vi "Intellirupter2.vi"() -> ()   [LabVIEW 2016]
uses:
  <vilib>/rvi/Emulation/niFpgaGetClockAttributes.vi
  <vilib>/rvi/Emulation/niFpgaSctlEmulationGetInTimedLoop.vi
  <vilib>/rvi/Emulation/niFpgaEmulationReportErrorSimple.vi
  <vilib>/rvi/eio/common/nirviEmuTemplateMethod_errors.vi
  <vilib>/rvi/interface/RandomDataEmulation/niFpgaRandomDataHandleErrors.vi
  <vilib>/rvi/Emulation/niFpgaCriticalErrorInLSC.vi
  <vilib>/eio/EIONode/EIONode.xnode
  <vilib>/rvi/DataTransferAndStorage/Container/XNode/niFpgaContainer.xnode
  <vilib>/rvi/interface/RandomDataEmulation/nirviRandomDataFpgaReadWriteTemplate.vi
panel:
  in  "Stop":bool
  in  "Loop Rate (uS)":u32
  out "Data FIFO Full":bool
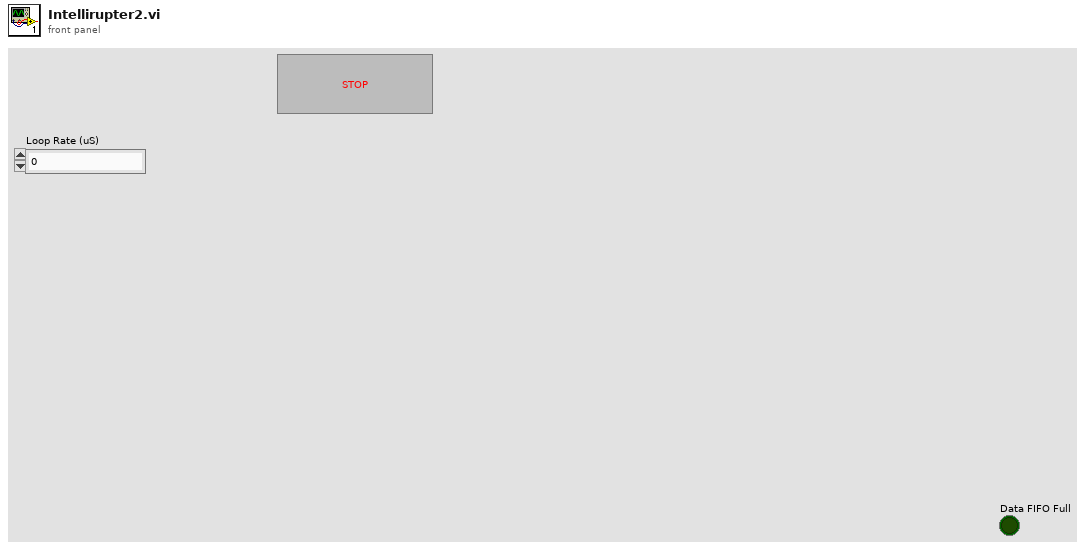
[diagram p1: front panel]
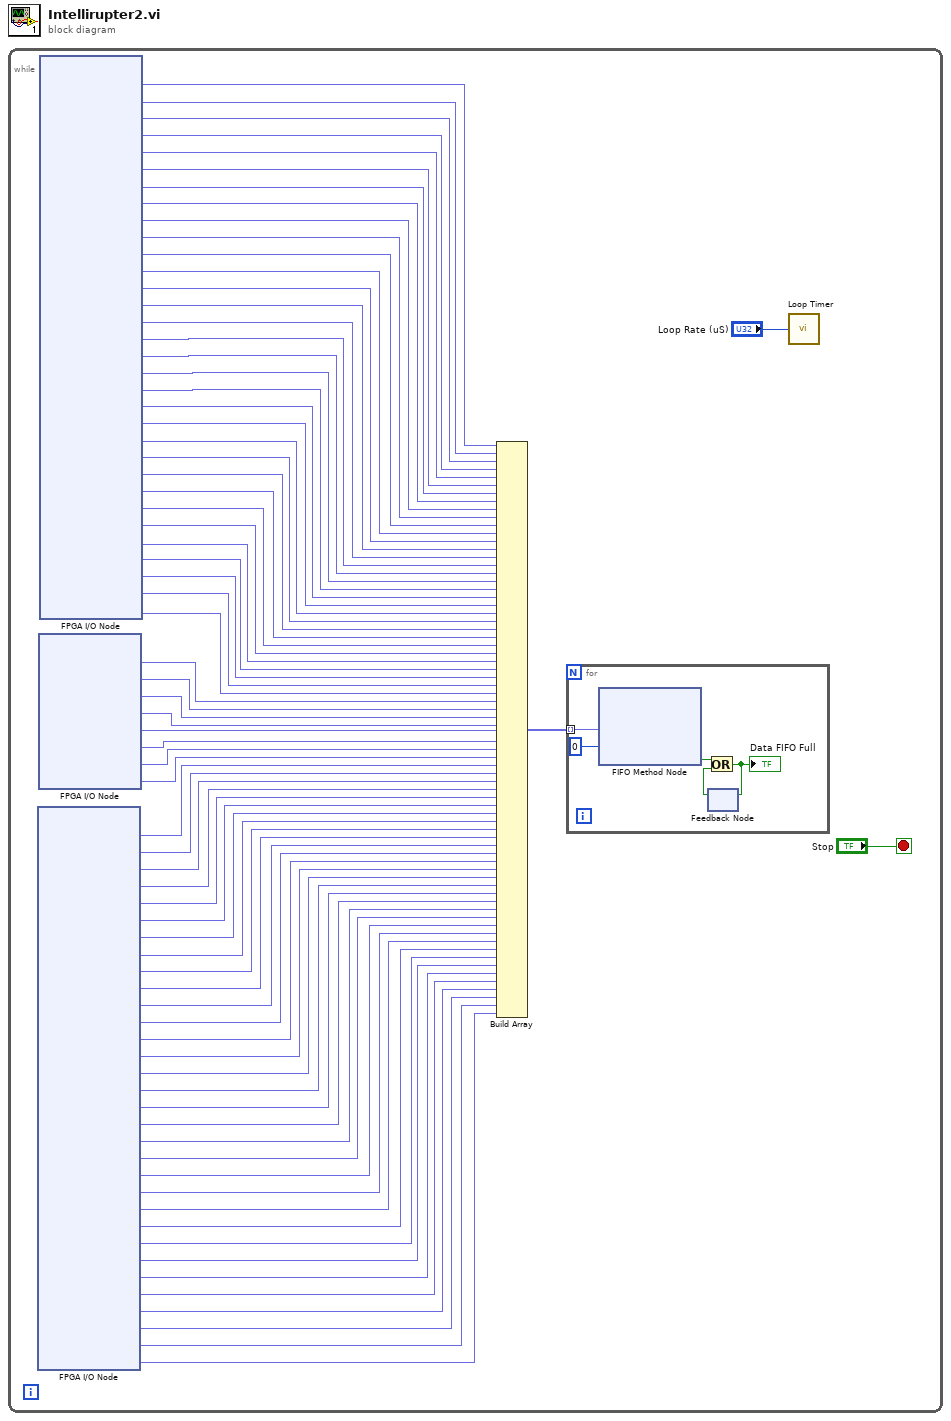
[diagram p0: block diagram]
diagram:
  n1 = while {
    stop <- "Stop" stop-if-true
    n2 = xnode "FPGA I/O Node"() -> ("Mod8/AI0"=w33:fxp<+/-,26,5>, "Mod8/AI1"=w32:fxp<+/-,26,5>, "Mod8/AI2"=w31:fxp<+/-,26,5>, "Mod8/AI3"=w30:fxp<+/-,26,5>, "Mod8/AI4"=w29:fxp<+/-,26,5>, "Mod8/AI5"=w28:fxp<+/-,26,5>, "Mod8/AI6"=w27:fxp<+/-,26,5>, "Mod8/AI7"=w26:fxp<+/-,26,5>, "Mod8/AI8"=w25:fxp<+/-,26,5>, "Mod8/AI9"=w24:fxp<+/-,26,5>, "Mod8/AI10"=w23:fxp<+/-,26,5>, "Mod8/AI11"=w22:fxp<+/-,26,5>, "Mod8/AI12"=w21:fxp<+/-,26,5>, "Mod8/AI13"=w20:fxp<+/-,26,5>, "Mod8/AI14"=w19:fxp<+/-,26,5>, "Mod8/AI15"=w18:fxp<+/-,26,5>, "Mod8/AI16"=w17:fxp<+/-,26,5>, "Mod8/AI17"=w16:fxp<+/-,26,5>, "Mod8/AI18"=w15:fxp<+/-,26,5>, "Mod8/AI19"=w14:fxp<+/-,26,5>, "Mod8/AI20"=w13:fxp<+/-,26,5>, "Mod8/AI21"=w12:fxp<+/-,26,5>, "Mod8/AI22"=w11:fxp<+/-,26,5>, "Mod8/AI23"=w10:fxp<+/-,26,5>, "Mod8/AI24"=w9:fxp<+/-,26,5>, "Mod8/AI25"=w8:fxp<+/-,26,5>, "Mod8/AI26"=w7:fxp<+/-,26,5>, "Mod8/AI27"=w6:fxp<+/-,26,5>, "Mod8/AI28"=w5:fxp<+/-,26,5>, "Mod8/AI29"=w4:fxp<+/-,26,5>, "Mod8/AI30"=w3:fxp<+/-,26,5>, "Mod8/AI31"=w2:fxp<+/-,26,5>)  [unwired: 32 in, 32 out]
    n3 = xnode "FPGA I/O Node"() -> ("Mod5/AI20"=w41:fxp<+/-,26,5>, "Mod5/AI1"=w40:fxp<+/-,26,5>, "Mod5/AI2"=w39:fxp<+/-,26,5>, "Mod5/AI3"=w38:fxp<+/-,26,5>, "Mod5/AI0"=w37:fxp<+/-,26,5>, "Mod5/AI21"=w36:fxp<+/-,26,5>, "Mod5/AI22"=w35:fxp<+/-,26,5>, "Mod5/AI23"=w34:fxp<+/-,26,5>)  [unwired: 8 in, 8 out]
    n4 = xnode "FPGA I/O Node"() -> ("Mod1/AI0"=w73:fxp<+/-,26,5>, "Mod1/AI1"=w72:fxp<+/-,26,5>, "Mod1/AI2"=w71:fxp<+/-,26,5>, "Mod1/AI3"=w70:fxp<+/-,26,5>, "Mod1/AI4"=w69:fxp<+/-,26,5>, "Mod1/AI5"=w68:fxp<+/-,26,5>, "Mod1/AI6"=w67:fxp<+/-,26,5>, "Mod1/AI7"=w66:fxp<+/-,26,5>, "Mod1/AI8"=w65:fxp<+/-,26,5>, "Mod1/AI9"=w64:fxp<+/-,26,5>, "Mod1/AI10"=w63:fxp<+/-,26,5>, "Mod1/AI11"=w62:fxp<+/-,26,5>, "Mod1/AI12"=w61:fxp<+/-,26,5>, "Mod1/AI13"=w60:fxp<+/-,26,5>, "Mod1/AI14"=w59:fxp<+/-,26,5>, "Mod1/AI15"=w58:fxp<+/-,26,5>, "Mod1/AI16"=w57:fxp<+/-,26,5>, "Mod1/AI17"=w56:fxp<+/-,26,5>, "Mod1/AI18"=w55:fxp<+/-,26,5>, "Mod1/AI19"=w54:fxp<+/-,26,5>, "Mod1/AI20"=w53:fxp<+/-,26,5>, "Mod1/AI21"=w52:fxp<+/-,26,5>, "Mod1/AI22"=w51:fxp<+/-,26,5>, "Mod1/AI23"=w50:fxp<+/-,26,5>, "Mod1/AI24"=w49:fxp<+/-,26,5>, "Mod1/AI25"=w48:fxp<+/-,26,5>, "Mod1/AI26"=w47:fxp<+/-,26,5>, "Mod1/AI27"=w46:fxp<+/-,26,5>, "Mod1/AI28"=w45:fxp<+/-,26,5>, "Mod1/AI29"=w44:fxp<+/-,26,5>, "Mod1/AI30"=w43:fxp<+/-,26,5>, "Mod1/AI31"=w42:fxp<+/-,26,5>)  [unwired: 32 in, 32 out]
    n5 = Build Array(w73, w72, w71, w70, w69, w68, w67, w66, w65, w64, w63, w62, w61, w60, w59, w58, w57, w56, w55, w54, w53, w52, w51, w50, w49, w48, w47, w46, w45, w44, w43, w42, w41, w40, w39, w38, w37, w36, w35, w34, w33, w32, w31, w30, w29, w28, w27, w26, w25, w24, w23, w22, w21, w20, w19, w18, w17, w16, w15, w14, w13, w12, w11, w10, w9, w8, w7, w6, w5, w4, w3, w2) -> (w1:fxp<+/-,26,5>[])
    n6 = for {
      tunnel: w1 -> [w78] mode=indexing
      n7 = xnode ("FIFO Method Node")("Element"=w78, "Timeout"=0) -> ("Timed Out?"=w76:bool)  [unwired: 1 in, 1 out]
      n8 = feedback #1() -> (w80:bool)  [unwired: 1 out]
      n9 = Or(x=w76, y=w80) -> (x .or. y?=w79:bool)
      "Data FIFO Full" <- w79
      n10 = feedback-in #1(w79) -> ()
    }
    n11 = call "Loop Timer"("Count(uSec)"="Loop Rate (uS)") -> ()  [unwired: 1 out]
  }
